vi "Test Complex Matrix Type.vi"(9 "relative tolerance":dbl=-1.0, 10 "matrix type":T1=10 items=["Hermitian Positive Definite"=10, "Hermitian Positive Semi-Definite"=11, "Symmetric"=20, "Hermitian"=21], 11 "Input Matrix":T2) -> (0 "error":i32, 3 "is type?":bool)   [LabVIEW 2020, in "NI_AALPro.lvlib"]
doc: "Tests whether<B> Input Matrix</B> is a matrix of special type. Wire data to the <B>Input Matrix</B> input to determine the polymorphic instance to use or manually select the instance."
uses:
  <vilib>/Analysis/NI_AALPro.lvlib
  <vilib>/Analysis/Matrix/Datatypes/ComplexMatrix.ctl
  <vilib>/Analysis/_algsub.llb/Complex Matrix Type for Test.ctl
  <vilib>/Analysis/Matrix/NI_Matrix.lvlib
panel:
  # "Test Matrix Type"
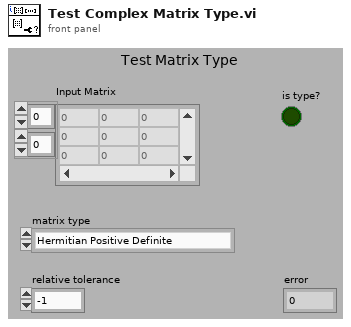
[diagram p1: front panel]
types:
  T1 = typedef "NI_AALPro.lvlib/Complex Matrix Type for Test.ctl" = i32
  T2 = typedef "NI_Matrix.lvlib/ComplexMatrix.ctl" = cdb[][]
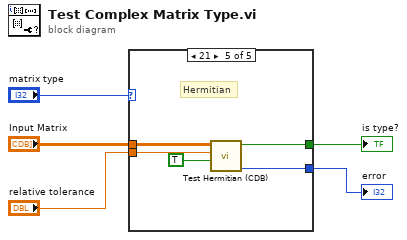
[diagram p0: block diagram]
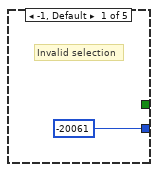
[diagram p2: hidden frame]
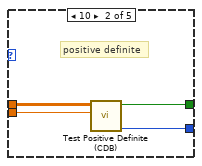
[diagram p3: hidden frame]
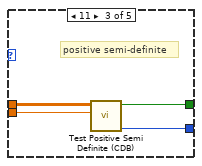
[diagram p4: hidden frame]
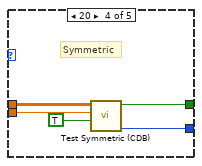
[diagram p5: hidden frame]
diagram:
  n1 = case shown="21" "matrix type" {
    tunnel: "Input Matrix" -> [_ w10 w14 w19 w24]
    tunnel: "relative tolerance" -> [_ w9 w13 w18 w23]
    tunnel: [_ w8 w11 w16 w21] -> w2
    tunnel: [-20061 ("return type") w7 w12 w17 w22] -> w1
    frame -1, Default {
      # "Invalid selection"
    }
    frame 10 {
      # "positive definite"
      n2 = call <vilib>:"Test Positive Definite (CDB).vi"("relative tolerance"=w9, "Input Matrix"=w10) -> ("error"=w7:i32, "positive definite?"=w8:bool)  [unwired: 8 out]
    }
    frame 11 {
      # "positive semi-definite"
      n3 = call <vilib>:"Test Positive Semi Definite (CDB).vi"("relative tolerance"=w13, "Input Matrix"=w14) -> ("error"=w12:i32, "positive semidefinite?"=w11:bool)  [unwired: 8 out]
    }
    frame 20 {
      # "Symmetric"
      n4 = call <vilib>:"Test Symmetric (CDB).vi"("relative tolerance?"=TRUE, "tolerance"=w18, "Input Matrix"=w19) -> ("error"=w17:i32, "Symmetric?"=w16:bool)  [unwired: 7 out]
    }
    frame 21 {
      # "Hermitian"
      n5 = call <vilib>:"Test Hermitian (CDB).vi"("relative tolerance?"=TRUE, "tolerance"=w23, "Input Matrix"=w24) -> ("error"=w22:i32, "Hermitian?"=w21:bool)  [unwired: 7 out]
    }
  }
  "error" <- w1
  "is type?" <- w2
